vi "Handle Mouse Down.vi"(4 "PlatMods":T2, 6 "Mods":cluster{"Double Click":bool, "Menu Key":bool}, 8 "error in (no error)":errorcluster, 9 "Button":u16, 10 "Coords":T3, 11 "Test Executive View in":refnum<class "Test Executive View.lvclass">) -> (0 "error out":errorcluster, 2 "Mouse Down Filtered Event Data":T1, 3 "Test Executive View out":refnum<class "Test Executive View.lvclass">)   [LabVIEW 2020, in "Test Executive View.lvclass"]
uses:
  <vilib>/gpm_packages/@cs/Test-executive-builder/Example/Application/Test Executive View/Test Executive View/Test Executive View.lvclass
  C:/Program Files/National Instruments/LabVIEW 2020/vi.lib/gpm_packages/@cs/Test-executive-builder/Source/Test Executive Builder View/Test Executive Builder View/Test Executive Builder View.lvclass
  <vilib>/Utility/miscctls.llb/LVPoint32TypeDef.ctl
  <vilib>/gpm_packages/@cs/Test-executive-builder/Source/Application Dependencies/Mouse Down Filtered Event Data.ctl
  <vilib>/gpm_packages/@cs/Test-executive-builder/Source/Test Executive Builder View/Test Executive Builder View/Test Executive Builder View.lvclass/Test Executive Builder View.ctl
  <vilib>/gpm_packages/@cs/Test-executive-builder/Source/Test Executive Builder View/Test Executive Builder View/Test Executive Builder View.lvclass
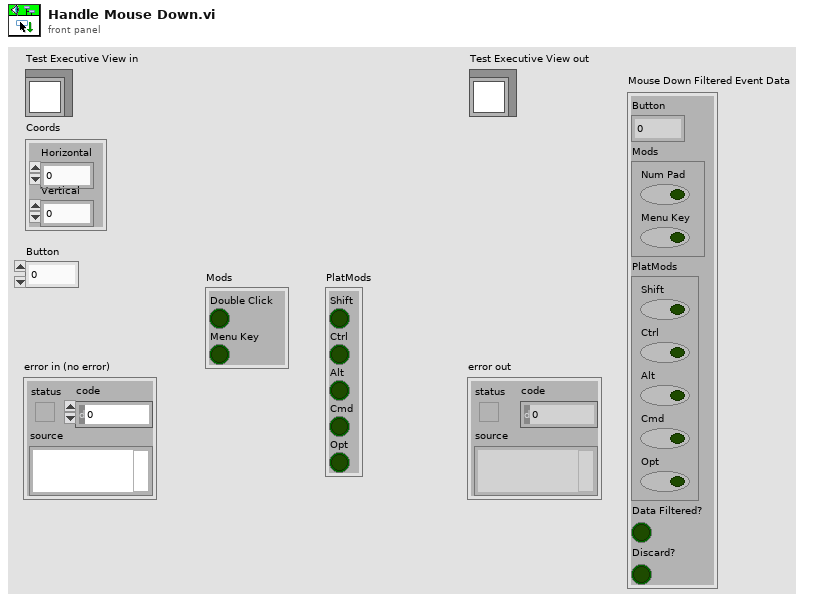
[diagram p1: front panel]
types:
  T1 = typedef "Mouse Down Filtered Event Data.ctl" = cluster{"Button":u16, "Mods":cluster{"Num Pad":bool, "Menu Key":bool}, "PlatMods":cluster{"Shift":bool, "Ctrl":bool, "Alt":bool, "Cmd":bool, "Opt":bool}, "Data Filtered?":bool, "Discard?":bool}
  T2 = cluster{"Shift":bool, "Ctrl":bool, "Alt":bool, "Cmd":bool, "Opt":bool}
  T3 = typedef "LVPoint32TypeDef.ctl" = cluster{"Horizontal":i32, "Vertical":i32}
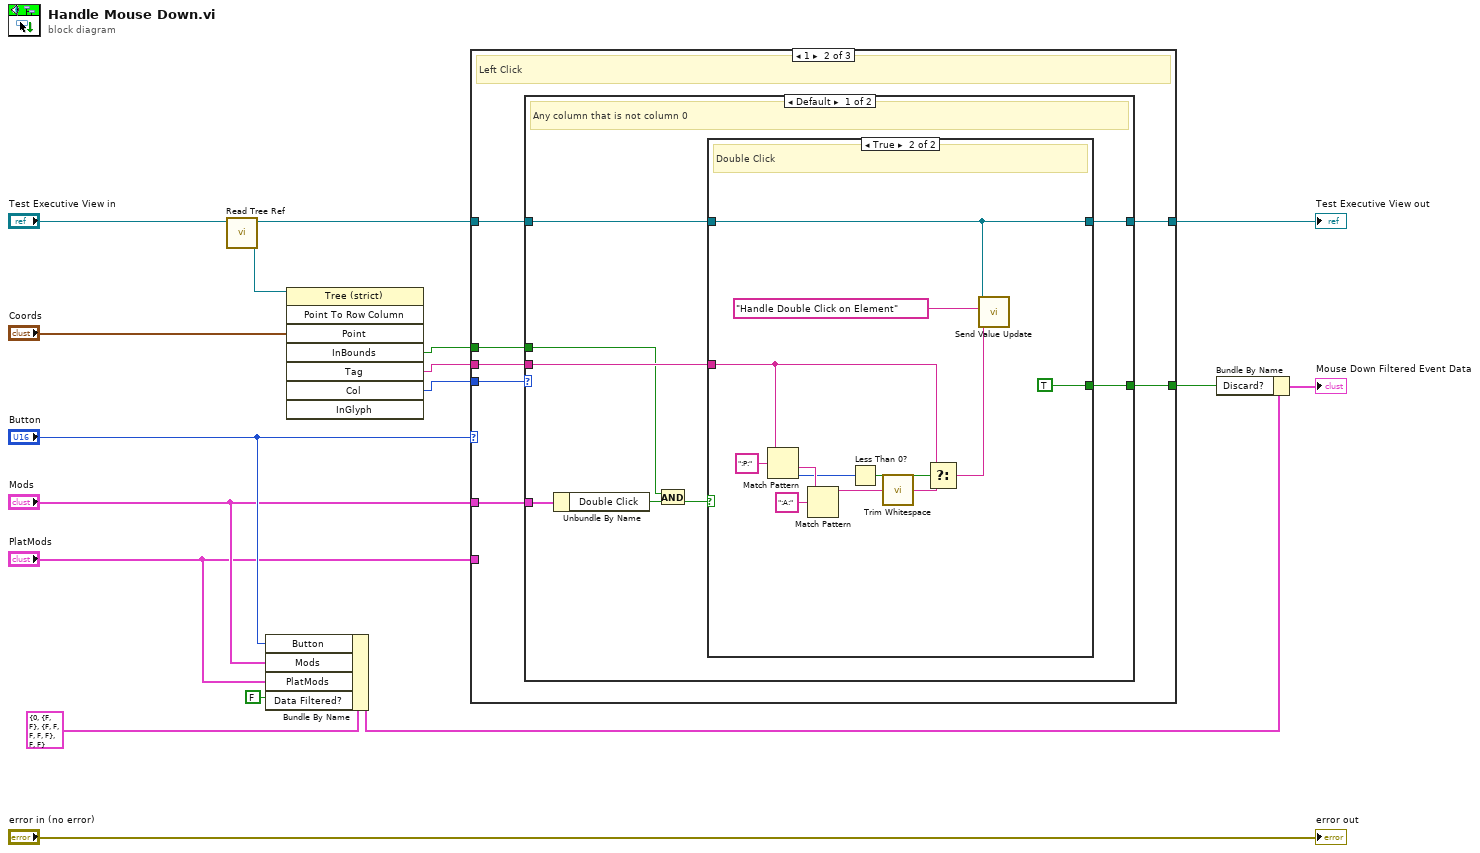
[diagram p0: block diagram]
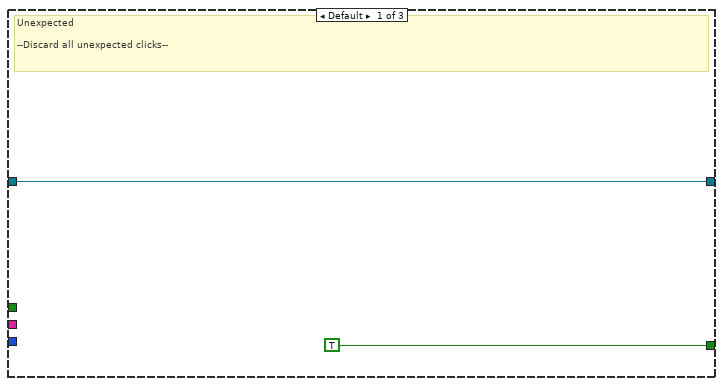
[diagram p2: hidden frame]
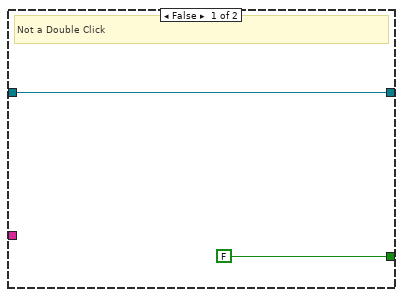
[diagram p3: hidden frame]
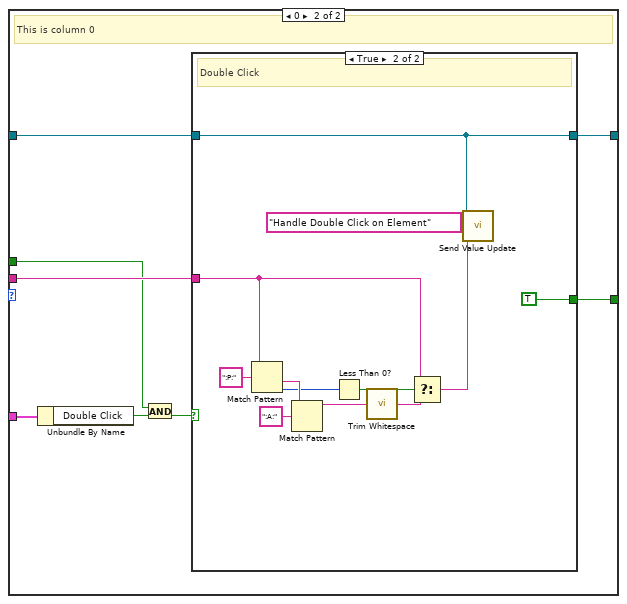
[diagram p4: hidden frame]
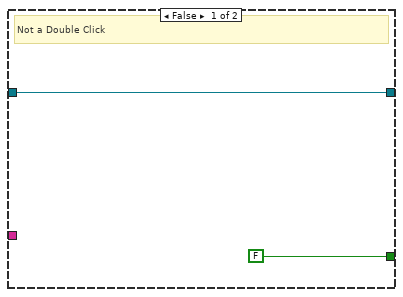
[diagram p5: hidden frame]
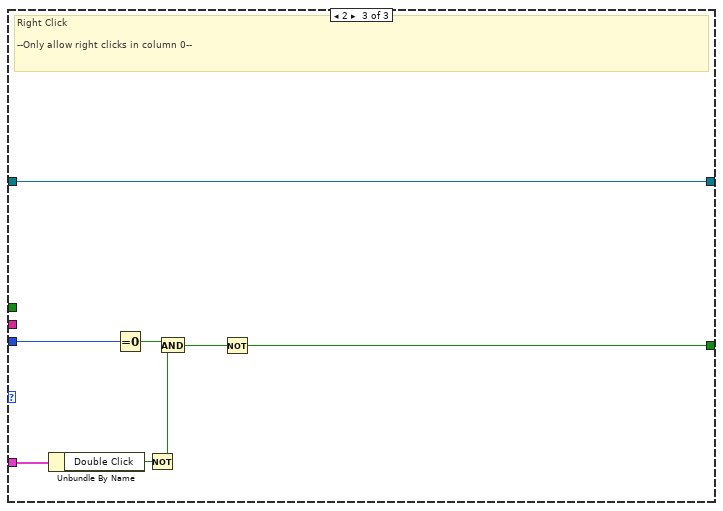
[diagram p6: hidden frame]
diagram:
  n1 = call <vilib>:"Read Tree Ref.vi"("Test Executive Builder View in"="Test Executive View in") -> ("Tree Ref"=w17:refnum<vi>, "Test Executive Builder View out"=w4:refnum<class "Test Executive View.lvclass">)  [unwired: 9 in]
  n2 = Bundle By Name(cluster=T1 {"Button"=0, "Mods"={"Num Pad"=FALSE, "Menu Key"=FALSE}, "PlatMods"={"Shift"=FALSE, "Ctrl"=FALSE, "Alt"=FALSE, "Cmd"=FALSE, "Opt"=FALSE}, "Data Filtered?"=FALSE, "Discard?"=FALSE} ("Mouse Down Filtered Event Data"), "Button"="Button", "Mods"="Mods", "PlatMods"="PlatMods", "Data Filtered?"=FALSE) -> (w8:T1)
  n3 = invoke class="Tree (strict)" method="Point To Row Column"(reference=w17, "Point"="Coords") -> ("InBounds"=w1:bool, "Tag"=w13:string, "Col"=w14:i32)  [unwired: 6 in, 5 out]
  n4 = case shown="1" "Button" {
    tunnel: w14 -> [_ w26 w78]
    tunnel: w13 -> [_ w21 _]
    tunnel: "Mods" -> [_ w25 w76]
    tunnel: "PlatMods" -> [_ _ _]
    tunnel: [TRUE w24 w72] -> w5
    tunnel: w4 -> [w18 w23 w71]
    tunnel: [w18 w22 w71] -> w3
    tunnel: w1 -> [_ w20 _]
    frame Default {
      # "Unexpected\n\n--Discard all unexpected clicks--"
    }
    frame 1 {
      # "Left Click"
      n5 = case shown="Default" w26 {
        tunnel: w25 -> [w34 w56]
        tunnel: [w32 w54] -> w24
        tunnel: w23 -> [w30 w52]
        tunnel: [w31 w53] -> w22
        tunnel: w21 -> [w29 w51]
        tunnel: w20 -> [w27 w49]
        frame Default {
          # "Any column that is not column 0"
          n6 = Unbundle By Name(w34) -> ("Double Click"=w33:bool)
          n7 = And(x=w27, y=w33) -> (x .and. y?=w28:bool)
          n8 = case shown="True" w28 {
            tunnel: [FALSE TRUE] -> w32
            tunnel: [w35 w39] -> w31
            tunnel: w30 -> [w35 w39]
            tunnel: w29 -> [_ w40]
            frame False {
              # "Not a Double Click"
            }
            frame True {
              # "Double Click"
              n9 = Match Pattern(string=w40, regular expression=":P:") -> (after substring=w46:string, offset past match=w45:i32)  [unwired: 1 in, 2 out]
              n10 = Match Pattern(string=w46, regular expression=":A:") -> (before substring=w44:string)  [unwired: 1 in, 3 out]
              n11 = Less Than 0?(x=w45) -> (x < 0?=w42:bool)
              n12 = call <vilib>:"Trim Whitespace.vi"("string"=w44) -> ("trimmed string"=w41:string)  [unwired: 1 in]
              n13 = Select(t=w40, s=w42, f=w41) -> (s? t:f=w38:string)
              n14 = call-dynamic "Send Value Update.vi"("Value"=w38, "Datum Name"="Handle Double Click on Element", "IViewable in"=w39) -> ()  [unwired: 8 in, 1 out]
            }
          }
        }
        frame 0 {
          # "This is column 0"
          n15 = Unbundle By Name(w56) -> ("Double Click"=w55:bool)
          n16 = And(x=w49, y=w55) -> (x .and. y?=w50:bool)
          n17 = case shown="True" w50 {
            tunnel: [FALSE TRUE] -> w54
            tunnel: [w57 w61] -> w53
            tunnel: w52 -> [w57 w61]
            tunnel: w51 -> [_ w62]
            frame False {
              # "Not a Double Click"
            }
            frame True {
              # "Double Click"
              n18 = Match Pattern(string=w62, regular expression=":P:") -> (after substring=w68:string, offset past match=w67:i32)  [unwired: 1 in, 2 out]
              n19 = Match Pattern(string=w68, regular expression=":A:") -> (before substring=w66:string)  [unwired: 1 in, 3 out]
              n20 = Less Than 0?(x=w67) -> (x < 0?=w64:bool)
              n21 = call <vilib>:"Trim Whitespace.vi"("string"=w66) -> ("trimmed string"=w63:string)  [unwired: 1 in]
              n22 = Select(t=w62, s=w64, f=w63) -> (s? t:f=w60:string)
              n23 = call-dynamic "Send Value Update.vi"("Value"=w60, "Datum Name"="Handle Double Click on Element", "IViewable in"=w61) -> ()  [unwired: 8 in, 1 out]
            }
          }
        }
      }
    }
    frame 2 {
      # "Right Click\n\n--Only allow right clicks in column 0--"
      n24 = Unbundle By Name(w76) -> ("Double Click"=w75:bool)
      n25 = Equal To 0?(x=w78) -> (x = 0?=w77:bool)
      n26 = Not(x=w75) -> (.not. x?=w74:bool)
      n27 = And(x=w77, y=w74) -> (x .and. y?=w73:bool)
      n28 = Not(x=w73) -> (.not. x?=w72:bool)
    }
  }
  "Test Executive View out" <- w3
  n29 = Bundle By Name(cluster=w8, "Discard?"=w5) -> (→"Mouse Down Filtered Event Data":T1)
  "error out" <- "error in (no error)"
